vi "Read Comm to gRPC.vi"(8 "error in (no error)":errorcluster, 11 "CIFPlugin in":refnum<class "Template_Plugin.lvclass">) -> (0 "error out":errorcluster, 3 "CIFPlugin out":refnum<class "Template_Plugin.lvclass">)   [LabVIEW 2021, in "Template_Plugin.lvclass"]
uses:
  Template_Plugin.lvclass
  Common/Typedef/OOB Comm/To gRPC Command Payload.ctl
  Common/Typedef/OOB Comm/To gRPC Command.ctl
  Common/Typedef/OOB Comm/To gRPC Command Data.ctl
  <vilib>/CIF Foundation/CIF CIPC/TypeDefs/Read Configuration.ctl
  <vilib>/CIF Foundation/CIF CIPC/TypeDefs/Read Position.ctl
  Template_Plugin.lvclass/Template_Plugin.ctl
  4f85eb37-057c-4128-a96e-b37296c04816.vi
  f031ee7a-4e36-46a2-9ecb-acdc30148a67.vi
  <vilib>/CIF Foundation/CIF CIPC/SubVIs/Wait For N Elements Available.vi
  <vilib>/CIF Foundation/CIF CIPC/SubVIs/Check Error.vi
  <vilib>/CIF Foundation/CIF CIPC/SubVIs/Get dll Path.vi
  <vilib>/CIF Foundation/CIF CIPC/SubVIs/Get Element Read Position.vi
  <vilib>/CIF Foundation/CIF CIPC/SubVIs/Set Element Read Position.vi
  <vilib>/CIF Foundation/CIF CIPC/SubVIs/Get Element Info Variant.vi
  <vilib>/Utility/error.llb/Trim Whitespace.vi
  <vilib>/Utility/error.llb/Error Cluster From Error Code.vi
  <vilib>/CIF Foundation/CIF CIPC/CIF_NI_CIPC.lvlib
  Common/Template_Common.lvlib
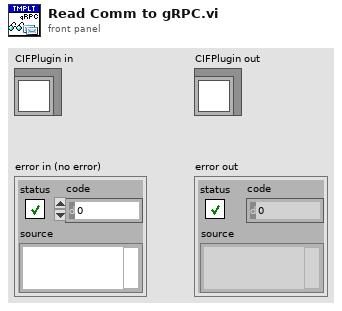
[diagram p1: front panel]
types:
  T1 = typedef "Template_Common.lvlib/To gRPC Command Payload.ctl" = cluster{"-> gRPC Command":T2, "-> gRPC Data":T3}
  T2 = typedef "Template_Common.lvlib/To gRPC Command.ctl" = enum16{"Read Data", "Read DVR Data"}
  T3 = typedef "Template_Common.lvlib/To gRPC Command Data.ctl" = cluster{"Cmd Data 1 -> gRPC":i32}
  T4 = typedef "CIF_NI_CIPC.lvlib/Read Configuration.ctl" = cluster{"Read Position":T5, "Element Offset":i32, "Prepend Array Size":bool, "Get Read Position":bool}
  T5 = typedef "CIF_NI_CIPC.lvlib/Read Position.ctl" = enum16{"Next", "Newest", "Oldest", "Next Available", "Absolute"}
  T6 = typedef "Template_Common.lvlib/To gRPC DVR Data.ctl" = cluster{"Data 1 DVR -> gRPC ":i32}
  T7 = typedef "Template_Common.lvlib/To gRPC Cyclic Data.ctl" = cluster{"Data 1 -> gRPC":i32, "Statistics":T8}
  T8 = typedef "Template_Plugin.lvclass/Statistics.ctl" = cluster{"Iterations":u64}
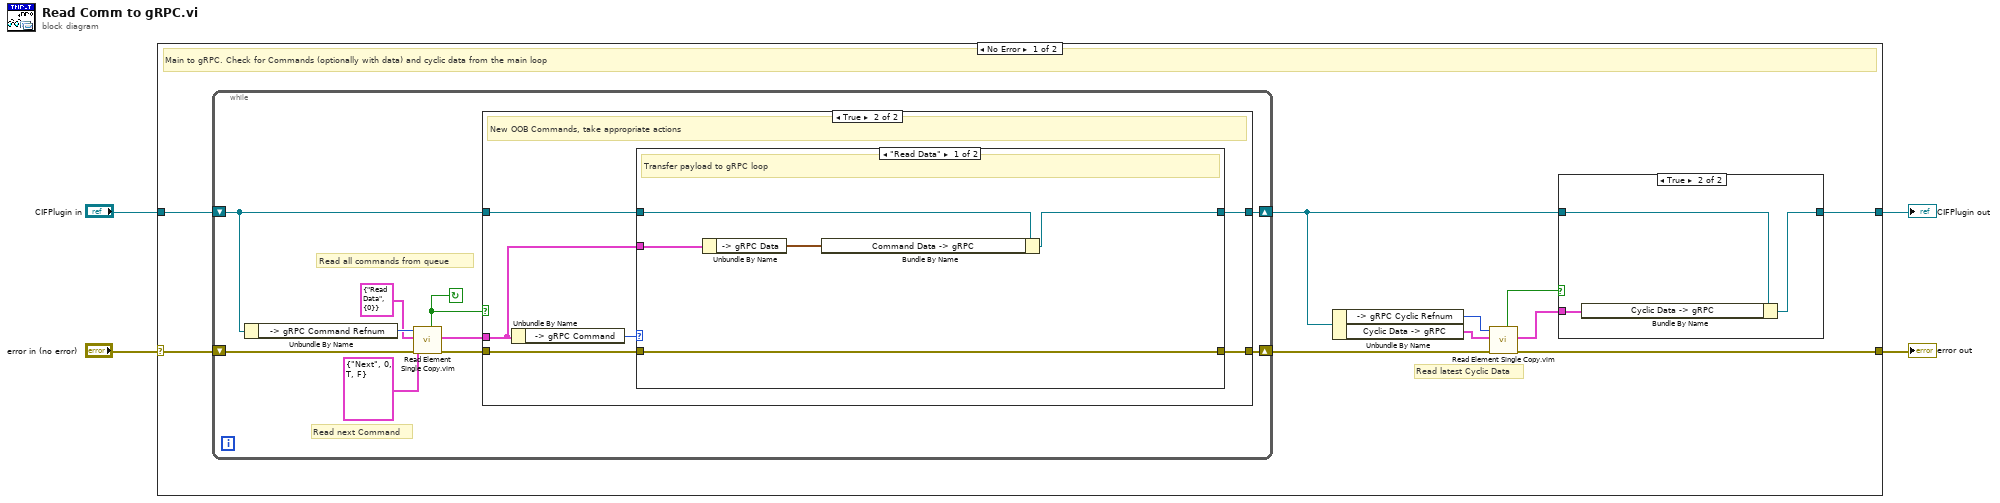
[diagram p0: block diagram]
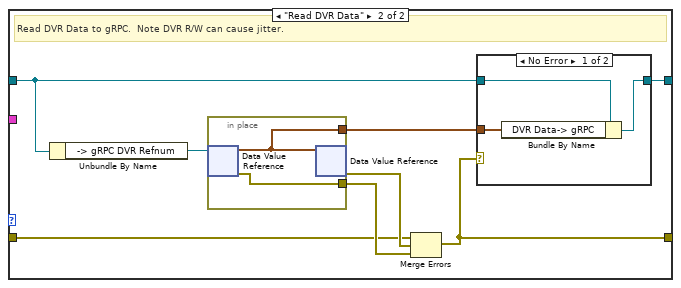
[diagram p3: hidden frame]
diagram:
  n1 = case shown="No Error" "error in (no error)" {
    selector: "error in (no error)" -> [w14 w57]
    tunnel: [w6 w57] -> w3
    tunnel: [w5 w56] -> w1
    tunnel: "CIFPlugin in" -> [w13 w56]
    frame No Error {
      # "Read latest Cyclic Data"
      # "Main to gRPC. Check for Commands (optionally with data) and cyclic data from the main loop"
      n2 = while {
        shift-right: [w19] -> w11
        shift-left: w14 -> [w23]
        shift-right: [w17] -> w7
        shift-left: w13 -> [w22]
        stop <- w15 continue-if-true
        # "Read all commands from queue"
        # "Read next Command"
        n3 = Unbundle By Name(w22) -> ("-> gRPC Command Refnum"=w24:u64)
        n4 = call "Read Element Single Copy.vim"("error in (no error)"=w23, "Read Configuration"=T4 {"Read Position"=enum."Next", "Element Offset"=0, "Prepend Array Size"=TRUE, "Get Read Position"=FALSE}, "Data in"=T1 {"-> gRPC Command"=enum."Read Data", "-> gRPC Data"={"Cmd Data 1 -> gRPC"=0}} ("-> gRPC Payload"), "CIPC Reference in"=w24) -> ("error out"=w21:errorcluster, "Data out"=w20:T1, "Success"=w15:bool)  [unwired: 3 in, 2 out]
        n5 = case shown="True" w15 {
          tunnel: w22 -> [w26 w32]
          tunnel: [w26 w27] -> w17
          tunnel: w21 -> [w25 w31]
          tunnel: [w25 w30] -> w19
          tunnel: w20 -> [_ w28]
          frame False {
            # "No new OOB Commands"
          }
          frame True {
            # "New OOB Commands, take appropriate actions"
            n6 = Unbundle By Name(w28) -> ("-> gRPC Command"=w29:T2)
            n7 = case shown="\"Read Data\"" w29 {
              tunnel: w31 -> [w37 w41]
              tunnel: w32 -> [w35 w40]
              tunnel: [w37 w38] -> w30
              tunnel: w28 -> [w36 _]
              tunnel: [w33 w39] -> w27
              frame "Read Data" {
                # "Transfer payload to gRPC loop"
                n8 = Unbundle By Name(w36) -> ("-> gRPC Data"=w34:T3)
                n9 = Bundle By Name(cluster=w35, "Command Data -> gRPC"=w34) -> (w33:refnum<class "Template_Plugin.lvclass">)
              }
              frame "Read DVR Data" {
                # "Read DVR Data to gRPC.  Note DVR R/W can cause jitter."
                n10 = Unbundle By Name(w40) -> ("-> gRPC DVR Refnum"=w43:refnum<data-value>)
                n11 = in-place {
                  in-place-border: [w51] -> w45
                  in-place-border: [w50] -> w42
                  n12 = in-place-dvr #1(w43) -> (w50:T6, w51:errorcluster)
                  n13 = in-place-dvr #1(w50) -> (w44:errorcluster)  [unwired: 1 out]
                }
                n14 = Merge Errors(w41, w44, w45) -> (w38:errorcluster)
                n15 = case shown="No Error" w38 {
                  tunnel: w42 -> [w48 _]
                  tunnel: w40 -> [w47 w49]
                  tunnel: [w46 w49] -> w39
                  frame No Error {
                    n16 = Bundle By Name(cluster=w47, "DVR Data-> gRPC"=w48) -> (w46:refnum<class "Template_Plugin.lvclass">)
                  }
                  frame Error {
                  }
                }
              }
            }
          }
        }
      }
      n17 = Unbundle By Name(w7) -> ("-> gRPC Cyclic Refnum"=w12:u64, "Cyclic Data -> gRPC"=w10:T7)
      n18 = call "Read Element Single Copy.vim"("error in (no error)"=w11, "Data in"=w10, "CIPC Reference in"=w12) -> ("error out"=w6:errorcluster, "Data out"=w8:T7, "Success"=w9:bool)  [unwired: 4 in, 2 out]
      n19 = case shown="True" w9 {
        tunnel: w8 -> [_ w54]
        tunnel: w7 -> [w52 w55]
        tunnel: [w52 w53] -> w5
        frame False {
        }
        frame True {
          n20 = Bundle By Name(cluster=w55, "Cyclic Data -> gRPC"=w54) -> (w53:refnum<class "Template_Plugin.lvclass">)
        }
      }
    }
    frame Error {
    }
  }
  "error out" <- w3
  "CIFPlugin out" <- w1
